vi "ps and atten.vi"() -> ()   [LabVIEW 2017]
panel:
  out "Attenuation":dbl
  out "PS":dbl
  out "Next step = True":bool
  out "i":i32
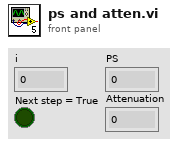
[diagram p1: front panel]
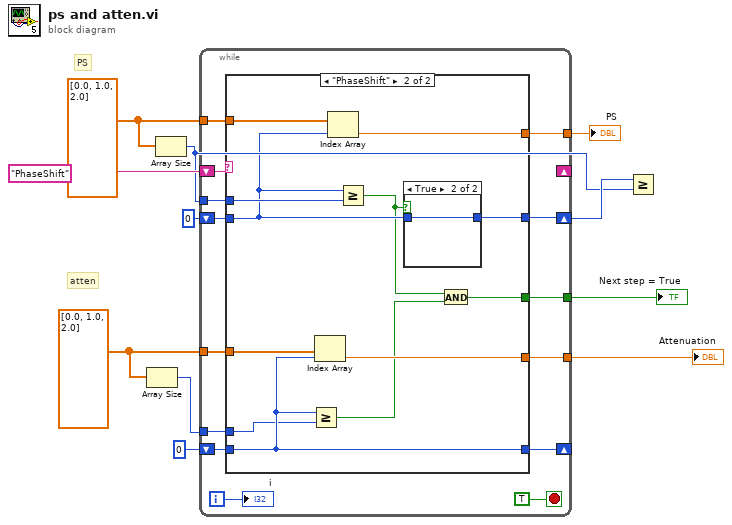
[diagram p0: block diagram]
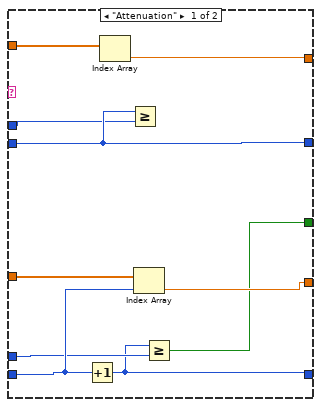
[diagram p2: hidden frame]
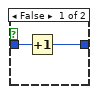
[diagram p3: hidden frame]
diagram:
  w8 = dbl[] [0.0, 1.0, 2.0]
  w10 = dbl[] [0.0, 1.0, 2.0]
  # "atten"
  # "PS"
  n1 = Array Size(array=w10) -> (size(s)=w9:i32)
  n2 = Array Size(array=w8) -> (size(s)=w1:i32)
  n3 = while {
    shift-right: [w15] -> _
    shift-left: 0 -> [w18]
    tunnel: w10 -> [w19]
    tunnel: w9 -> [w17]
    shift-right: [w23] -> w2
    shift-left: 0 -> [w22]
    tunnel: w8 -> [w21]
    tunnel: w1 -> [w24]
    shift-right: _ -> [_]
    shift-left: "PhaseShift" -> [w20]
    tunnel: [w16] -> w5
    tunnel: [w14] -> w4
    tunnel: [w13] -> w3
    i -> [w25]
    stop <- TRUE stop-if-true
    n4 = case shown="\"PhaseShift\"" w20 {
      tunnel: w24 -> [w26 w47]
      tunnel: [w27 w46] -> w23
      tunnel: w22 -> [w27 w42]
      tunnel: w21 -> [w32 w45]
      tunnel: w19 -> [w35 w43]
      tunnel: w18 -> [w34 w41]
      tunnel: w17 -> [w33 w40]
      tunnel: [w31 w44] -> w16
      tunnel: [w29 w41] -> w15
      tunnel: [w30 w39] -> w14
      tunnel: [w28 w37] -> w13
      frame "Attenuation" {
        n5 = Increment(x=w34) -> (x+1=w29:i32)
        n6 = Index Array(array=w32) -> (element=w31:dbl)  [unwired: 1 in]
        n7 = Greater Or Equal?(x=w27, y=w26) -> ()  [unwired: 1 out]
        n8 = Index Array(array=w35, index=w34) -> (element=w30:dbl)
        n9 = Greater Or Equal?(x=w29, y=w33) -> (x >= y?=w28:bool)
      }
      frame "PhaseShift" {
        n10 = Greater Or Equal?(x=w41, y=w40) -> (x >= y?=w38:bool)
        n11 = Index Array(array=w43, index=w41) -> (element=w39:dbl)
        n12 = Index Array(array=w45, index=w42) -> (element=w44:dbl)
        n13 = Greater Or Equal?(x=w42, y=w47) -> (x >= y?=w36:bool)
        n14 = case shown="True" w36 {
          tunnel: [w49 w50] -> w46
          tunnel: w42 -> [w48 w50]
          frame False {
            n15 = Increment(x=w48) -> (x+1=w49:i32)
          }
          frame True {
          }
        }
        n16 = And(x=w36, y=w38) -> (x .and. y?=w37:bool)
      }
    }
    "i" <- w25
  }
  "Next step = True" <- w3
  "PS" <- w5
  "Attenuation" <- w4
  n17 = Greater Or Equal?(x=w2, y=w1) -> ()  [unwired: 1 out]
